vi "HomeFGV.vi"(0 "Énum":enum16{"set", "get"}(ring), 1 "Booléen":bool) -> (7 "home ?":bool)   [LabVIEW 2020]
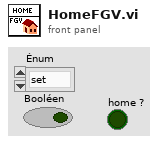
[diagram p1: front panel]
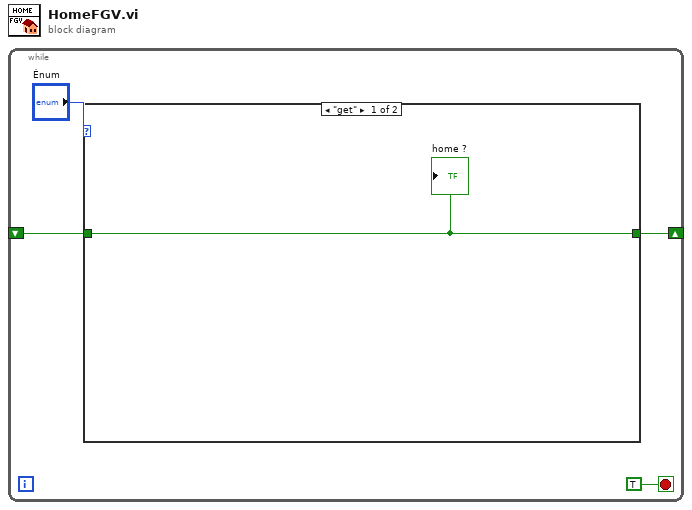
[diagram p0: block diagram]
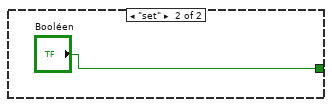
[diagram p2: hidden frame]
diagram:
  n1 = while {
    shift-right: [w2] -> _
    shift-left: _ -> [w1]
    stop <- TRUE stop-if-true
    n2 = case shown="\"get\"" "Énum" {
      tunnel: [w5 "Booléen"] -> w2
      tunnel: w1 -> [w5 _]
      frame "get" {
        "home ?" <- w5
      }
      frame "set" {
      }
    }
  }
